vi "Read DB.vi"(8 "error in (no error)":errorcluster, 11 "Configuration Database Actor in":refnum<class "Configuration Database Actor.lvclass">) -> (0 "error out":errorcluster, 3 "Configuration Database Actor out":refnum<class "Configuration Database Actor.lvclass">)   [LabVIEW 2019, in "Configuration Database Actor.lvlib" / "Configuration Database Actor.lvclass"]
uses:
  Configuration Database Actor.lvclass
  C:/Program Files (x86)/National Instruments/LabVIEW 2019/vi.lib/ActorFramework/Actor/Actor.lvclass
  <vilib>/ActorFramework/Actor/Actor.lvclass/Actor.ctl
  Configuration Database Actor.lvclass/Configuration Database Actor.ctl
  Record Data -Cluster.ctl
  Elevator Controller/Elevator Controller Messages/Get DB Record Msg/Get DB Record Msg.lvclass/Get DB Record Msg.ctl
  <vilib>/ActorFramework/Message Enqueuer/Message Enqueuer.lvclass/Message Enqueuer.ctl
  <vilib>/ActorFramework/Message Enqueuer/Enqueue.vi
  Elevator Controller/Elevator Controller Messages/Get DB Record Msg/Get DB Record Msg.lvclass
  C:/Program Files (x86)/National Instruments/LabVIEW 2019/vi.lib/ActorFramework/Message/Message.lvclass
  <vilib>/ActorFramework/Message Priority Queue/Priority Enqueue.vi
  <vilib>/ActorFramework/Actor/Actor.lvclass
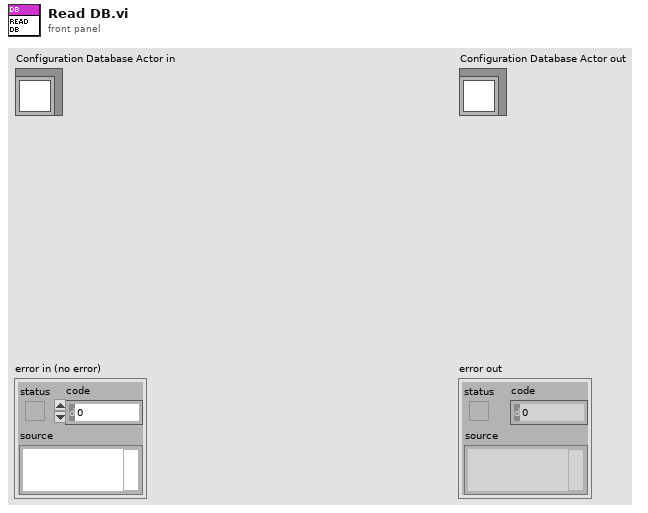
[diagram p1: front panel]
types:
  T1 = typedef "Configuration Database Actor.lvlib/Configuration Database Actor.lvclass/Record Data -Cluster.ctl" = cluster{"Door Open":dbl, "Door Close":dbl, "Travel Time":dbl, "Inactivity Time":dbl}
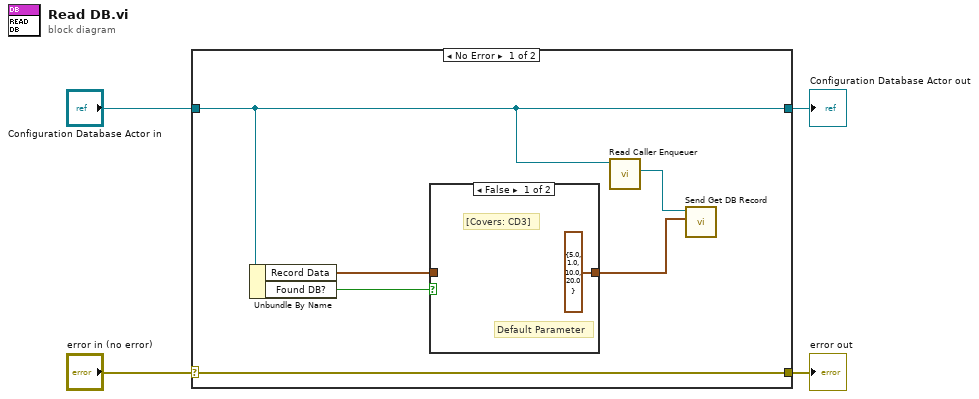
[diagram p0: block diagram]
diagram:
  n1 = case shown="No Error" "error in (no error)" {
    selector: "error in (no error)" -> [w10 w14]
    tunnel: [w10 w14] -> w3
    tunnel: [w9 w13] -> w1
    tunnel: "Configuration Database Actor in" -> [w9 w13]
    frame No Error {
      n2 = Unbundle By Name(w9) -> ("Record Data"=w7:T1, "Found DB?"=w5:bool)
      n3 = case shown="False" w5 {
        tunnel: w7 -> [_ w12]
        tunnel: [T1 {"Door Open"=5.0, "Door Close"=1.0, "Travel Time"=10.0, "Inactivity Time"=20.0} ("Record Data") w12] -> w6
        frame False {
          # "[Covers: CD3]"
          # "Default Parameter"
        }
        frame True {
        }
      }
      n4 = call <vilib>:"Read Caller Enqueuer.vi"("Actor"=w9) -> ("Caller Enqueuer"=w8:refnum<class "Message Enqueuer.lvclass">)  [unwired: 10 in]
      n5 = call "Send Get DB Record.vi"("Record Data"=w6, "Message Enqueuer"=w8) -> ()  [unwired: 8 in, 2 out]
    }
    frame Error {
    }
  }
  "error out" <- w3
  "Configuration Database Actor out" <- w1
